vi "Set Scopes.vi"(8 "error in (no error)":errorcluster, 10 "Scopes":string[](array[string]), 11 "OAuth2 in":refnum<class "OAuth2.lvclass">) -> (0 "error out":errorcluster, 3 "OAuth2 out":refnum<class "OAuth2.lvclass">)   [LabVIEW 2020, in "OAuth2.lvlib" / "OAuth2.lvclass"]
uses:
  OAuth2.lvclass
  Request/Request.lvclass
  5f682dac-2761-4b67-ab78-6fb3d1f9eafd.vi
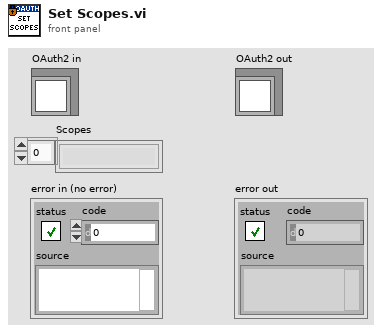
[diagram p1: front panel]
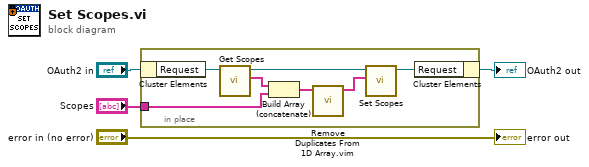
[diagram p0: block diagram]
diagram:
  n1 = in-place {
    in-place-border: "Scopes" -> [w7]
    n2 = in-place-cluster #1("OAuth2 in") -> ("Request"=w11:refnum<class "Request.lvclass">)
    n3 = call "Get Scopes.vi"("Request in"=w11) -> ("Scopes"=w8:string[], "Request out"=w9:refnum<class "Request.lvclass">)  [unwired: 8 in, 1 out]
    n4 = Build Array (concatenate)(w8, w7) -> (w6:string[])
    n5 = call "Remove Duplicates From 1D Array.vim"("array"=w6) -> ("array with duplicates removed"=w5:string[])  [unwired: 10 in]
    n6 = call "Set Scopes.vi"("Scopes"=w5, "Request in"=w9) -> ("Request out"=w10:refnum<class "Request.lvclass">)  [unwired: 8 in, 1 out]
    n7 = in-place-cluster #1("Request"=w10) -> (→"OAuth2 out":refnum<class "OAuth2.lvclass">)
  }
  "error out" <- "error in (no error)"
